vi "check if lines are same type.vi"(8 "error in":errorcluster, 11 "Lines in":T2[](array[typedef])) -> (0 "error out":errorcluster, 1 "type":T1, 2 "all same type?":bool, 3 "Lines out":T2[](array[typedef]))   [LabVIEW 2014, in "Shared Memory configuration.lvclass"]
uses:
  Shared Memory configuration.lvclass
  Line.ctl
  <vilib>/NI/Tag Bus Module Framework/channel/TBM channel.lvclass
  <vilib>/NI/Tag Bus/tag/Data Type.ctl
  <vilib>/NI/Tag Bus/tag/tag descriptor.lvclass/tag descriptor.ctl
  <vilib>/NI/Tag Bus/tag/tag descriptor.lvclass
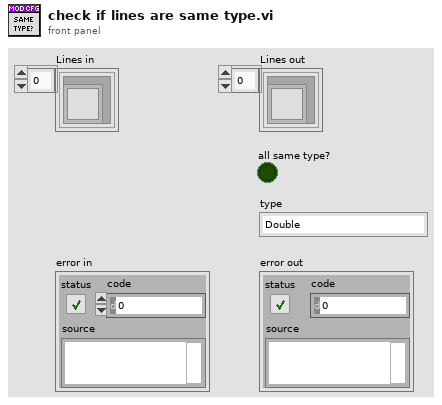
[diagram p1: front panel]
types:
  T1 = typedef "tag bus.lvlib/tag descriptor.lvclass/Data Type.ctl" = enum16{"Double", "Single", "I64", "I32", "I16", "I8", "U64", "U32", "U16", "U8", "Boolean", "String", "Array of Double", "Array of Single", "Array of I64", "Array of I32", "Array of I16", "Array of I8", "Array of U64", "Array of U32", "Array of U16", "Array of U8", "Array of Boolean", "Array of String"}
  T2 = typedef "Shared Memory configuration.lvclass/Line.ctl" = cluster{"channel":refnum<class "TBM channel.lvclass">}
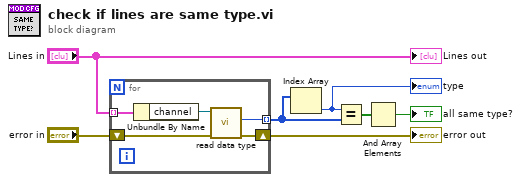
[diagram p0: block diagram]
diagram:
  n1 = for {
    tunnel: "Lines in" -> [w12] mode=indexing
    tunnel: [w10] -> w7 mode=indexing
    shift-right: [w8] -> w3
    shift-left: "error in" -> [w9]
    n2 = Unbundle By Name(w12) -> ("channel"=w11:refnum<class "TBM channel.lvclass">)
    n3 = call <vilib>:"read data type.vi"("error in"=w9, "system tag in"=w11) -> ("error out"=w8:errorcluster, "data type"=w10:T1)  [unwired: 7 in, 1 out]
  }
  "error out" <- w3
  n4 = Index Array(array=w7) -> (element=w1:T1)  [unwired: 1 in]
  "type" <- w1
  n5 = Equal?(x=w1, y=w7) -> (x = y?=w6:bool[])
  n6 = And Array Elements(Boolean array=w6) -> (logical AND=→"all same type?":bool)
  "Lines out" <- "Lines in"
